vi "Gmsg_PS_Publisher.vi"() -> ()   [LabVIEW 2015]
uses:
  source/actor/Publisher/FTW-Publisher.lvclass
panel:
  in  "Socket Type":enum16{"LabVIEW Queue", "TCP"}(ring)
  in  "OK Button":bool
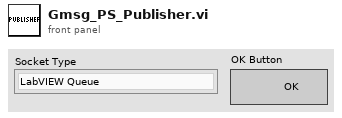
[diagram p1: front panel]
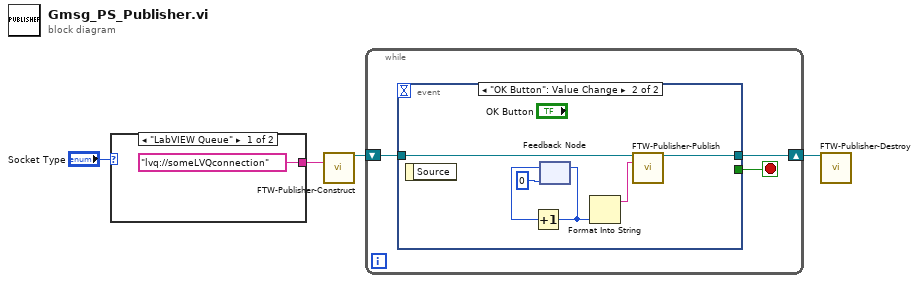
[diagram p0: block diagram]
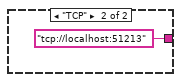
[diagram p2: hidden frame]
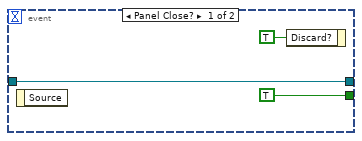
[diagram p3: hidden frame]
diagram:
  n1 = case shown="\"LabVIEW Queue\"" "Socket Type" {
    tunnel: ["lvq://someLVQconnection" "tcp://localhost:51213"] -> w2
    frame "LabVIEW Queue" {
    }
    frame "TCP" {
    }
  }
  n2 = call "FTW-Publisher-Construct.vi"("Address"=w2) -> ("FTW-Publisher Out"=w4:refnum<class "FTW-Publisher.lvclass">)  [unwired: 12 in, 2 out]
  n3 = while {
    shift-right: [w7] -> w3
    shift-left: w4 -> [w8]
    stop <- w9 stop-if-true
    n4 = event shown="[1] \"OK Button\": Value Change" {
      selector: _ -> [_ _]
      dyn-events: _ -> [_ _]
      timeout: _ -> [_ _]
      tunnel: [TRUE _] -> w9
      tunnel: w8 -> [w10 w16]
      tunnel: [w10 w15] -> w7
      event Panel Close? {
        n5 = event-data() -> ()  [unwired: 1 in, 1 out]
        n6 = event-data("Discard?"=TRUE) -> ()  [unwired: 1 in, 1 out]
      }
      event "OK Button": Value Change {
        n7 = event-data() -> ()  [unwired: 1 in, 1 out]
        n8 = feedback #1(0) -> (w17:i32)
        n9 = Increment(x=w17) -> (x+1=w14:i32)
        n10 = feedback-in #1(w14) -> ()
        n11 = Format Into String(w14) -> (resulting string=w13:string)  [unwired: 3 in, 1 out]
        n12 = call "FTW-Publisher-Publish.vi"("FTW-Publisher In"=w16, "Header"=w13) -> ("FTW-Publisher Out"=w15:refnum<class "FTW-Publisher.lvclass">)  [unwired: 12 in, 1 out]
      }
    }
  }
  n13 = call "FTW-Publisher-Destroy.vi"("FTW-Publisher In"=w3) -> ()  [unwired: 14 in, 1 out]
